vi "T7MOD_Read_INT32_Register.vi"(8 "error in":errorcluster, 9 "LabJack INT32 Register":i32=55122, 10 "Remote Port":u16=502, 11 "Remote IP Address":string="192.168.1.15") -> (0 "error out":errorcluster, 1 "Read At":timestamp, 2 "Raw Data Read":u16[](array[numeric]), 3 "Read INT32":i32)   [LabVIEW 2015]
uses:
  Serial Link Layer/NI_Modbus_Cleaned/NI Modbus121Clean.llb/MB Ethernet Master Query Read Input Registers (poly).vi
panel:
  # "Output"
  # "TCP Parameters"
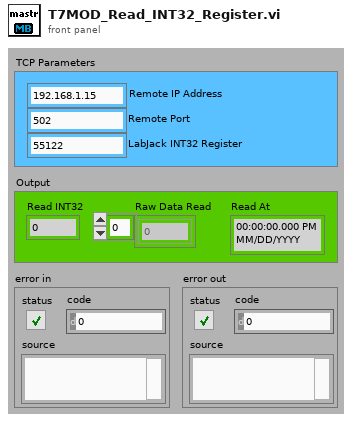
[diagram p1: front panel]
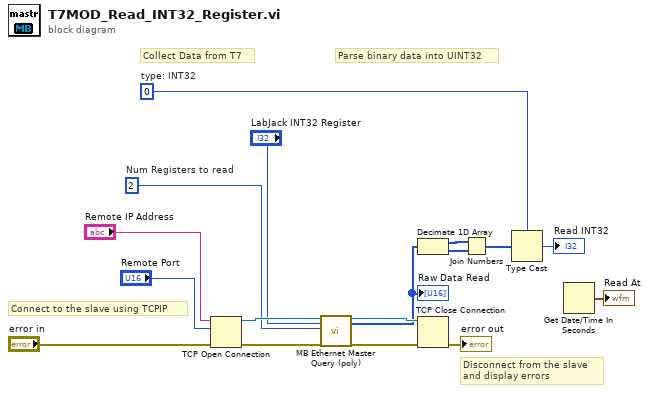
[diagram p0: block diagram]
diagram:
  w3 = 0  # type: INT32
  w10 = 2  # Num Registers to read
  # "Parse binary data into UINT32"
  # "Collect Data from T7"
  # "Disconnect from the slave\nand display errors"
  # "Connect to the slave using TCPIP"
  n1 = TCP Open Connection(address="Remote IP Address", remote port or service name="Remote Port", error in (no error)="error in") -> (connection ID=w15:refnum<k5>, error out=w14:errorcluster)  [unwired: 2 in]
  n2 = call-poly "MB Ethernet Master Query (poly).vi"("TCP Connection Refnum in"=w15, "Starting Address"="LabJack INT32 Register", "Quantity"=w10, "error in"=w14) -> ("TCP Connection Refnum (dup)"=w12:refnum<k5>, "Input Registers"=w5:u16[], "error out"=w13:errorcluster)  [unwired: 12 in, 1 out]
  "Raw Data Read" <- w5
  n3 = Decimate 1D Array(w5) -> (w7:u16[], w6:u16[])
  n4 = TCP Close Connection(connection ID=w12, error in (no error)=w13) -> (error out=→"error out":errorcluster)  [unwired: 2 out]
  n5 = Join Numbers(hi=w7, lo=w6) -> ((hi.lo)=w4:u32[])
  n6 = Type Cast(type=w3, x=w4) -> (*(type *) &x=→"Read INT32":i32)
  n7 = Get Date/Time In Seconds() -> (seconds since 1Jan1904=→"Read At":timestamp)
